vi "读取配置文件引用.vi"(8 "error in (no error)":errorcluster caption="错误输入（无错误）", 11 "启动器输入":refnum<class "启动器.lvclass">) -> (0 "error out":errorcluster caption="错误输出", 2 "config data":T1 caption="配置数据", 3 "启动器输出":refnum<class "启动器.lvclass">)   [LabVIEW 2017, in "启动器.lvlib" / "启动器.lvclass"]
doc: "获取配置文件引用, 如果引用无效则报错."
uses:
  <vilib>/Utility/config.llb/Config Data RefNum.ctl
  <vilib>/Utility/config.llb/NI_LVConfig.lvlib
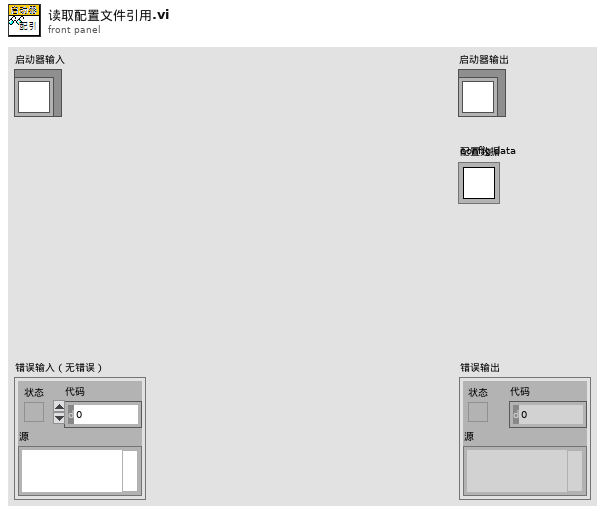
[diagram p1: front panel]
types:
  T1 = typedef "NI_LVConfig.lvlib/Config Data RefNum.ctl" = refnum<k1>
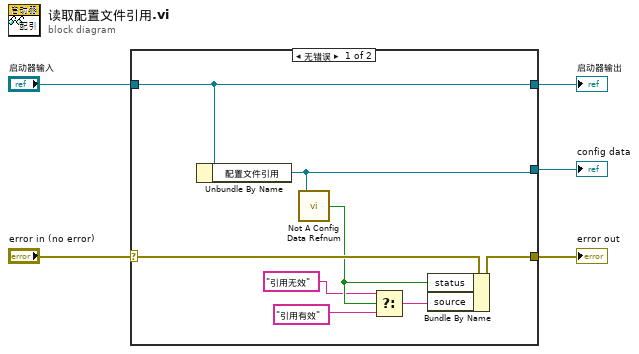
[diagram p0: block diagram]
diagram:
  n1 = case shown="无错误" "error in (no error)" {
    selector: "error in (no error)" -> [w13 w14]
    tunnel: [w10 w14] -> w4
    tunnel: [w12 w15] -> w2
    tunnel: "启动器输入" -> [w12 w15]
    tunnel: [w11 _] -> w1
    frame No Error {
      n2 = Unbundle By Name(w12) -> ("配置文件引用"=w11:T1)
      n3 = call <vilib>:"Not A Config Data Refnum.vi"("refnum"=w11) -> ("not a config data refnum"=w9:bool)
      n4 = Select(t="引用无效", s=w9, f="引用有效") -> (s? t:f=w6:string)
      n5 = Bundle By Name(cluster=w13, "status"=w9, "source"=w6) -> (w10:errorcluster)
    }
    frame Error {
    }
  }
  "error out" <- w4
  "启动器输出" <- w2
  "config data" <- w1
